vi "save_file.vi"(7 "Data":dbl[](array[numeric]), 8 "error in (no error)":errorcluster, 10 "Yes/No":bool, 11 "File Type":T1) -> (0 "error out":errorcluster)   [LabVIEW 2024]
uses:
  controls/file_type.ctl
  <vilib>/Utility/TDMS File Viewer/NI_TDMS File Viewer.lvlib
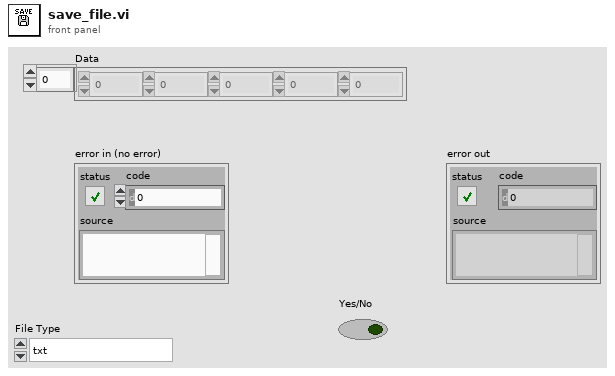
[diagram p1: front panel]
types:
  T1 = typedef "file_type.ctl" = enum16{"txt", "csv", "tdms"}
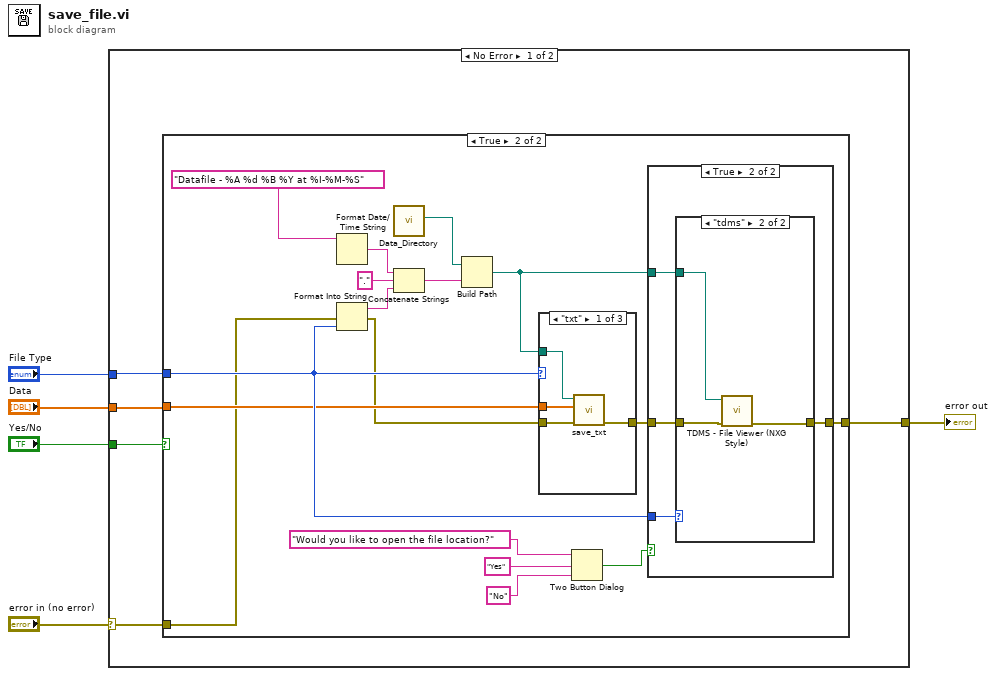
[diagram p0: block diagram]
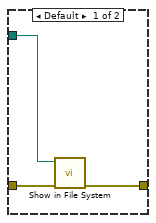
[diagram p4: hidden frame]
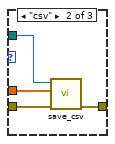
[diagram p5: hidden frame]
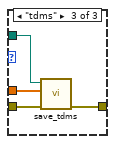
[diagram p6: hidden frame]
diagram:
  n1 = case shown="No Error" "error in (no error)" {
    selector: "error in (no error)" -> [w10 w52]
    tunnel: "Data" -> [w7 _]
    tunnel: [w9 w52] -> w3
    tunnel: "File Type" -> [w8 _]
    tunnel: "Yes/No" -> [w6 _]
    frame No Error {
      n2 = case shown="True" w6 {
        tunnel: w8 -> [_ w22]
        tunnel: w7 -> [_ w20]
        tunnel: [w11 w17] -> w9
        tunnel: w10 -> [w11 w16]
        frame False {
        }
        frame True {
          n3 = Format Date/Time String(time format string (%c)="Datafile - %A %d %B %Y at %I-%M-%S") -> (date/time string=w27:string)  [unwired: 2 in]
          n4 = Format Into String(error in=w16, w22) -> (resulting string=w25:string, error out=w19:errorcluster)  [unwired: 2 in]
          n5 = call "Data_Directory.vi"() -> ("Data Directory"=w21:path)  [unwired: 11 in]
          n6 = Concatenate Strings(w27, "." ("string"), w25) -> (w24:string)
          n7 = Build Path(base path=w21, name or relative path=w24) -> (appended path=w23:path)
          n8 = case shown="\"txt\"" w22 {
            tunnel: w23 -> [w42 w47 w51]
            tunnel: w20 -> [w43 w46 w50]
            tunnel: w19 -> [w41 w45 w49]
            tunnel: [w40 w44 w48] -> w18
            frame "txt" {
              n9 = call "save_txt.vi"("error in (no error)"=w41, "Data"=w43, "Path"=w42) -> ("error out"=w40:errorcluster)  [unwired: 8 in]
            }
            frame "csv" {
              n10 = call "save_csv.vi"("error in (no error)"=w45, "Data"=w46, "Path"=w47) -> ("error out"=w44:errorcluster)  [unwired: 8 in]
            }
            frame "tdms" {
              n11 = call "save_tdms.vi"("error in (no error)"=w49, "Data"=w50, "Path"=w51) -> ("error out"=w48:errorcluster)  [unwired: 8 in]
            }
          }
          n12 = Two Button Dialog(message="Would you like to open the file location?", 1:"No" ("F button name (\"Cancel\")"), 2:"Yes" ("T button name (\"OK\")")) -> (T button?=w12:bool)
          n13 = case shown="True" w12 {
            tunnel: w23 -> [_ w32]
            tunnel: w22 -> [_ w33]
            tunnel: w18 -> [w29 w31]
            tunnel: [w29 w30] -> w17
            frame False {
            }
            frame True {
              n14 = case shown="\"tdms\"" w33 {
                tunnel: w32 -> [w34 w37]
                tunnel: w31 -> [w36 w39]
                tunnel: [w35 w38] -> w30
                frame Default {
                  n15 = call <vilib>:"Show in File System.vi"("error in (no error)"=w36, "file or directory path"=w34) -> ("error out"=w35:errorcluster)  [unwired: 9 in]
                }
                frame "tdms" {
                  n16 = call <vilib>:"TDMS - File Viewer (NXG Style).vi"("error in"=w39, "file in"=w37) -> ("error out"=w38:errorcluster)  [unwired: 8 in, 1 out]
                }
              }
            }
          }
        }
      }
    }
    frame Error {
    }
  }
  "error out" <- w3
